vi "Pressure Monitor GUI.vi"(9 "Standalone":bool=TRUE, 10 "Init Data":variant, 11 "My Name":string) -> ()   [LabVIEW 2021]
uses:
  typedefs/CC enum Operation Mode.ctl
  Subsystems/SS typedef cluster Instrument Command Queue Data.ctl
  Subsystems/SS cluster Data Queue type.ctl
  hk-channel-class/HK Item/HK Item.lvclass
  CryoCooler/Cryo Cooler/CryoCoolerAVC/CryoCoolerAVC Command cluster.ctl
  CryoCooler/Cryo Cooler/CryoCoolerAVC/CryoCoolerAVC Command enum.ctl
  Pressure Monitor/Pressure Monitor.lvclass
  typedefs/CC cluster Alarm Data.ctl
  Pressure Monitor/CC cluster Pressure Monitor Settings.ctl
  Pressure Monitor/Lesker Pressure/Lesker Pressure.lvclass
  C:/Development/prime/Prime-RIMAS/Pressure Monitor/Pressure Monitor/Pressure Monitor.lvclass
  Pressure Monitor/Pressure Monitor.lvclass/Pressure Monitor.ctl
  hk-channel-class/HK Item/HK Item.lvclass/HK Item.ctl
  hk-channel-class/HK Item/HK Channel cluster Telemetry Data.ctl
  hk-channel-class/HK Item/HK Channel enum Data Type.ctl
  <vilib>/Utility/error.llb/DialogType.ctl
  Pressure Monitor/Lesker Pressure/Lesker Pressure.lvclass/Lesker Pressure.ctl
  hk-channel-class/HK Item/Write Source.vi
panel:
  in  "Mode":T1
  in  "Tab Control":enum32{"Pressure Monitor", "Engineering", "Log"}(tab)
  in  "Reconnect":bool
  in  "Clear History":bool
  in  "Log Scale":bool=TRUE
  out "Alarm Message":string
  out "Pressure Connected":bool
  out "Alarm":bool
  in  "Status":i32[](listbox) caption="Pressure Monitor"
  out "XY Graph":T2(graph)
  in  "Inst Filament":bool caption="Filament"
  in  "Pump Filament":bool
  in  "Pressure Alarm Level":dbl format="%^_3g"
  in  "Enable Pump Reading?":bool
  in  "Pump Lesker Addr":refnum<visa-resource-name>
  in  "Instrument Lesker Addr":refnum<visa-resource-name>
  in  "CryoCooler Type":u16(ring) items=["Simulation", "PRIME"]
  in  "Close":bool
  out "Log":string
  # "Guage type is 392\nIf the Ion Gauge commands to turn the filament ON and OFF returns a SYNTAX Error, then you\nneed to go to the gauge front panel menu and select:\nFirst TURN IG OFF, then\nSETUP UNIT > IG CNTL > Set to RS485\n\nSee page 30 of the manual"
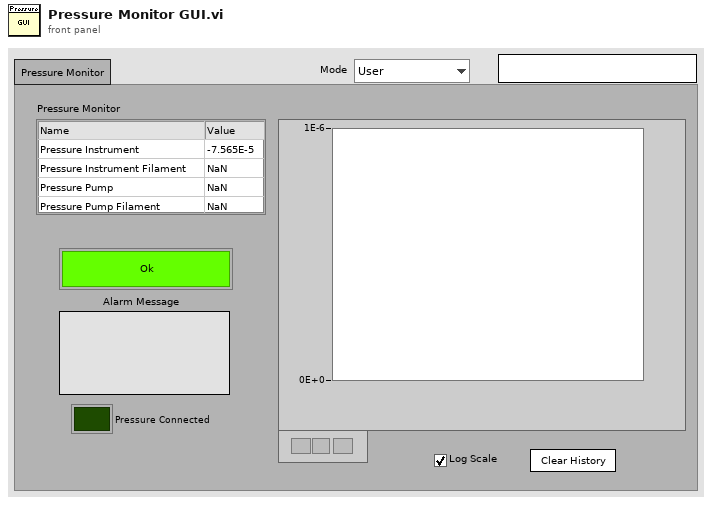
[diagram p1: front panel]
types:
  T1 = typedef "CC enum Operation Mode.ctl" = enum16{"User", "Engineering"}
  T2 = cluster{cluster{"Time Stamp":timestamp, "Numeric":dbl}[]}[]
  T3 = typedef "SS typedef cluster Instrument Command Queue Data.ctl" = cluster{"Cmd":string, "Parameters":variant}
  T4 = typedef "CryoCoolerAVC Command cluster.ctl" = cluster{"Command":T5, "Options":string, "Cryo Idx":i32}
  T5 = typedef "CryoCoolerAVC Command enum.ctl" = u16
  T6 = typedef "CC cluster Alarm Data.ctl" = cluster{"Measured Value":dbl, "Alarm Low":dbl, "Alarm High":dbl, "Message":string, "Source":string}
  T7 = typedef "CC cluster Pressure Monitor Settings.ctl" = cluster{"Lesker Addrs":refnum<visa-resource-name>[], "Enabled?":bool[], "Pressure Alarm Level":dbl, "Filaments":bool[]}
  T8 = cluster{"state":refnum<user-event>, "cmd q":refnum<queue>, "Cmd":T3, "Data Q":refnum<queue>, "error":errorcluster, "next poll":timestamp, "My Name":string, "poll":bool, "Channel List":refnum<class "HK Item.lvclass">[], "Focus Pos":dbl, "Data":dbl[], "Cryo Cmd":T4, "Alarm":bool, "PM Ref":refnum<class "Pressure Monitor.lvclass">, "Alarms":T6[], "Source":string, "Settings":T7}
  T9 = typedef "SS cluster Data Queue type.ctl" = cluster{"Source":string, "Type":string, "Data":variant}
  T10 = typedef "HK Item.lvclass/HK Channel enum Data Type.ctl" = enum16{"Floating Point", "Integer", "Enum", "String", "Waveform", "File"}
  T11 = typedef "HK Item.lvclass/HK Channel cluster Telemetry Data.ctl" = cluster{"Ch Names":string[], "Ch Values":dbl[], "Timestamp":timestamp, "Data Type":T10}
  T12 = typedef "CC cluster Device Index.ctl" = cluster{"Device Type Name":string, "Curr Device Name":string, "All Instances":string[]}
  T13 = cluster{"Select Ch":i32[], "Default Device":string}
  T14 = typedef "HK Item.lvclass/HK Channel Units and Setup.ctl" = cluster{"Unit Type":string, "Units":string, "Configuration":string, "Digits":i32, "Data Type":T10, "Exponential?":bool, "Source":string}
  T15 = cluster{cluster{"Time Stamp":timestamp, "Numeric":dbl}[]}
  T16 = typedef "DialogType.ctl" = u16
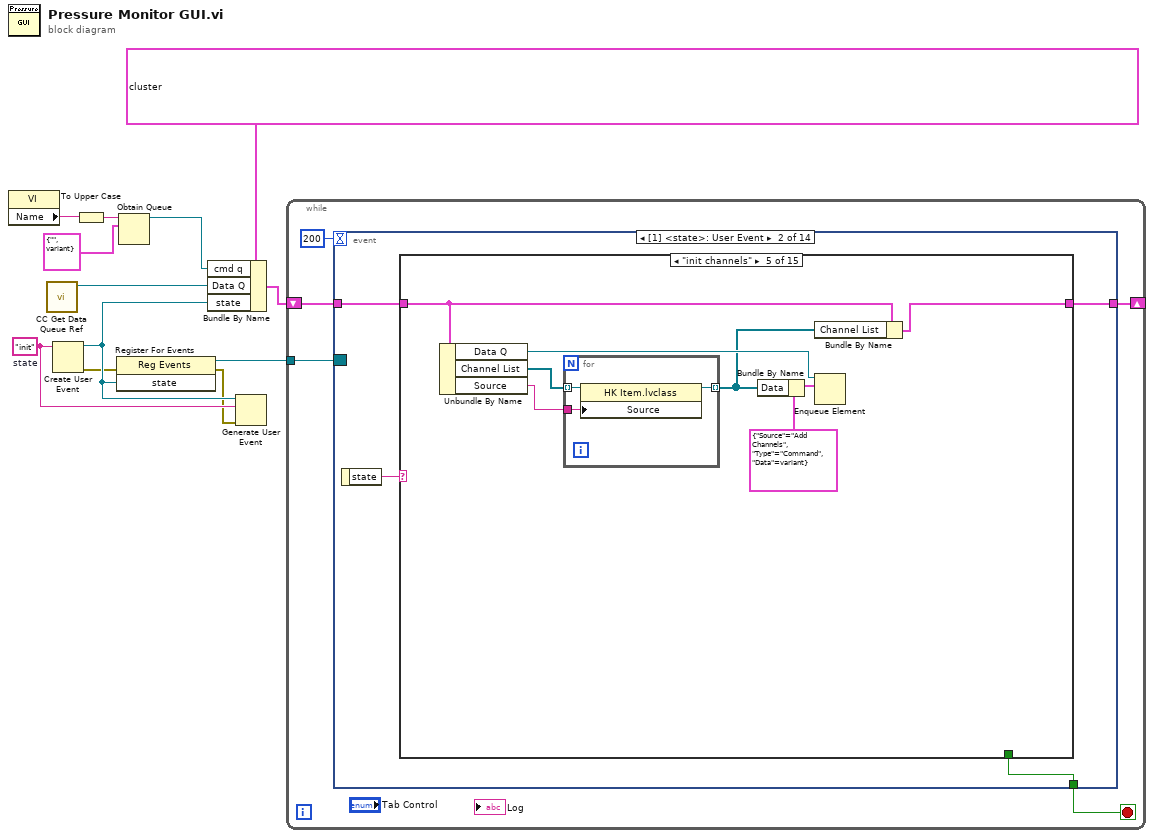
[diagram p0: block diagram]
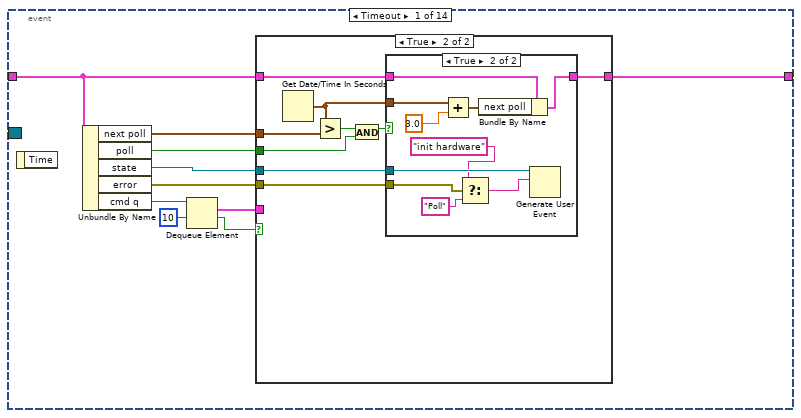
[diagram p2: hidden frame]
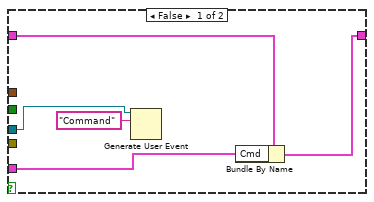
[diagram p3: hidden frame]
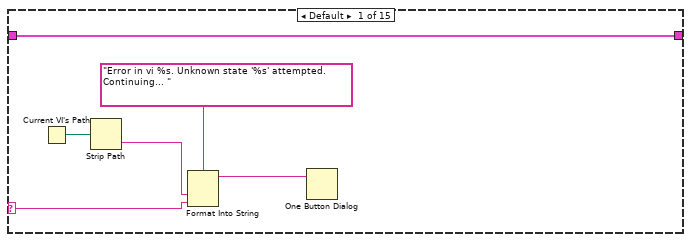
[diagram p5: hidden frame]
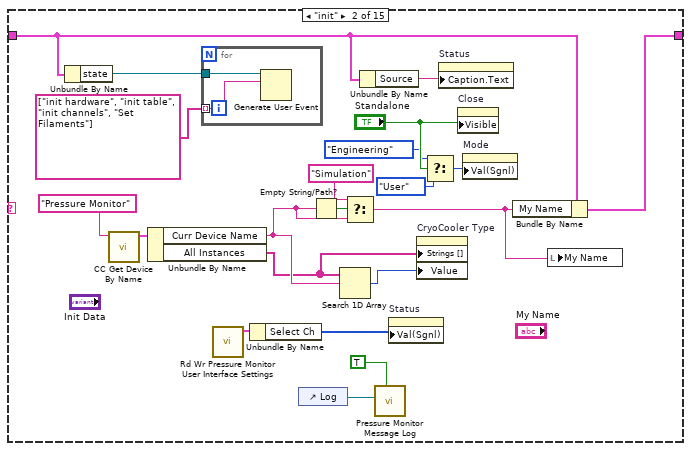
[diagram p6: hidden frame]
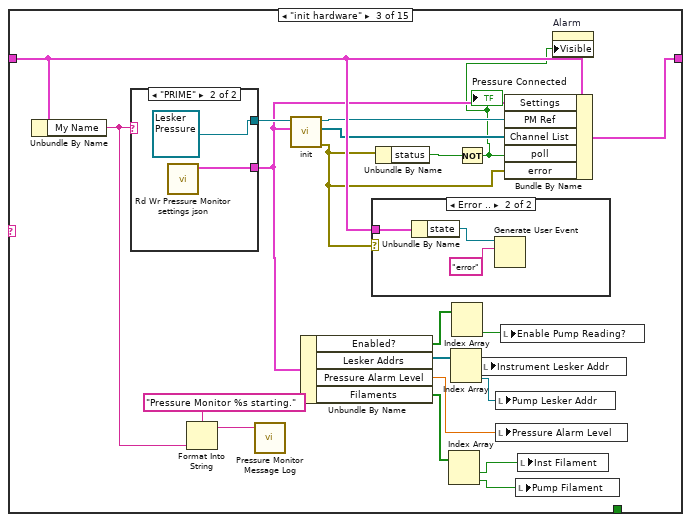
[diagram p7: hidden frame]
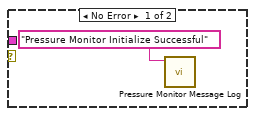
[diagram p8: hidden frame]
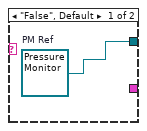
[diagram p9: hidden frame]
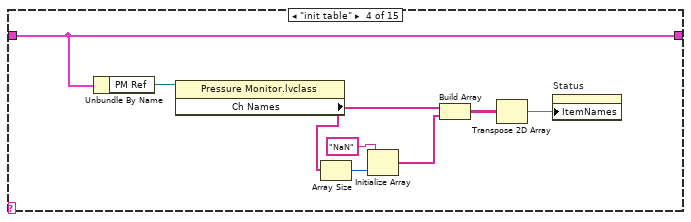
[diagram p10: hidden frame]
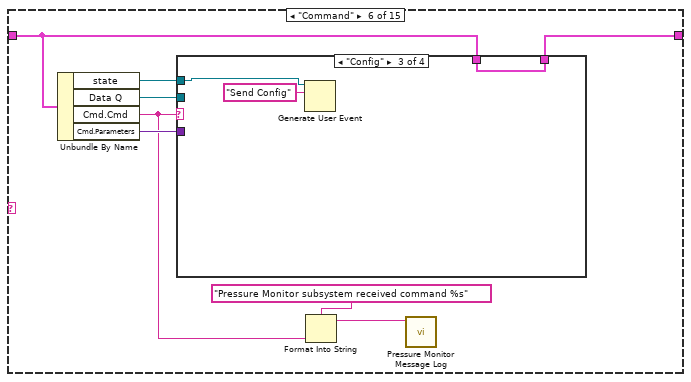
[diagram p11: hidden frame]
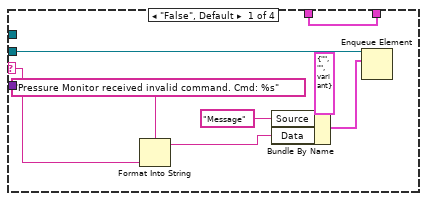
[diagram p12: hidden frame]
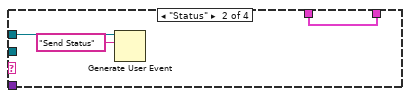
[diagram p13: hidden frame]
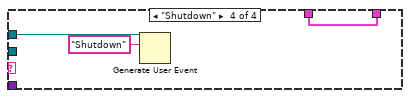
[diagram p14: hidden frame]
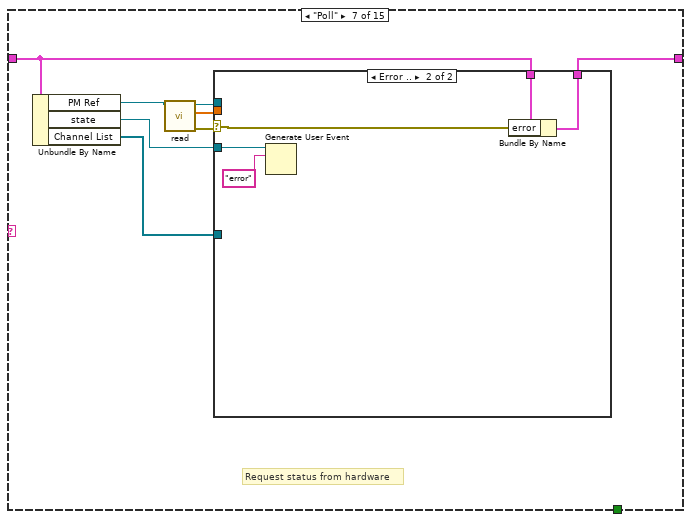
[diagram p15: hidden frame]
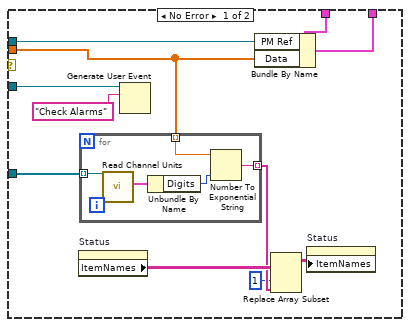
[diagram p16: hidden frame]
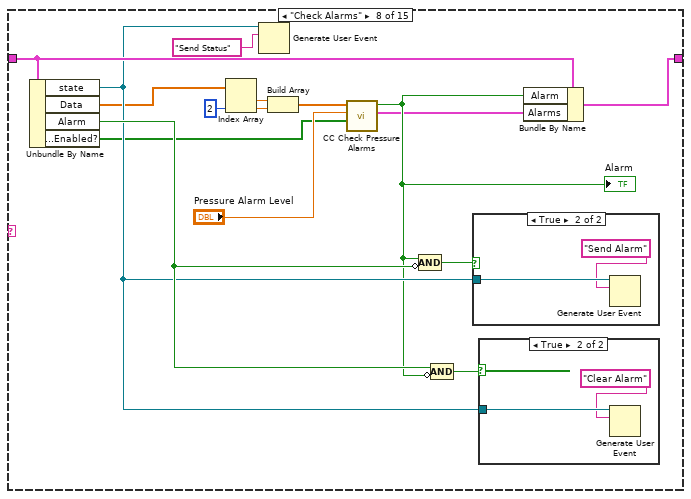
[diagram p17: hidden frame]
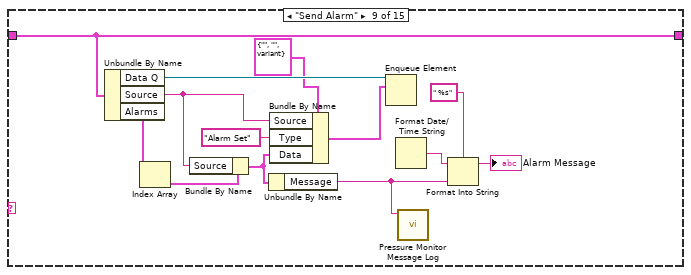
[diagram p20: hidden frame]
diagram:
  w8 = "init"  # state
  n1 = property class="VI"() -> ("Name"=w4:string)  [unwired: 2 in, 2 out]
  n2 = call "CC Get Data Queue Ref.vi"() -> ("Data Q"=w5:refnum<queue>)  [unwired: 10 in, 1 out]
  n3 = Create User Event(user event datatype=w8) -> (user event=w10:refnum<user-event>, error out=w6:errorcluster)  [unwired: 1 in]
  n4 = To Upper Case(1:w4) -> (0:w3:string)
  n5 = register-events(error in=w6, w10) -> (reference out=w9:refnum<event-registration>, error out=w7:errorcluster)  [unwired: 1 in]
  n6 = Obtain Queue(name (unnamed)=w3, element data type=T3 {"Cmd"="", "Parameters"=variant}) -> (queue out=w1:refnum<queue>)  [unwired: 3 in, 2 out]
  n7 = Bundle By Name(cluster=T8 {"state"=refnum, "cmd q"=refnum, "Cmd"={"Cmd"="", "Parameters"=variant}, "Data Q"=refnum, "error"={"status"=FALSE, "code"=0, "source"=""}, "next poll"=timestamp(0 s since 1904-01-01), "My Name"="", "poll"=FALSE, "Channel List"=[], "Focus Pos"=0.0, "Data"=[], "Cryo Cmd"={"Command"=0, "Options"="", "Cryo Idx"=0}, "Alarm"=FALSE, "PM Ref"=refnum, "Alarms"=[], "Source"="Pressure Monitor", "Settings"={"Lesker Addrs"=[], "Enabled?"=[], "Pressure Alarm Level"=0.0001, "Filaments"=[]}}, "cmd q"=w1, "Data Q"=w5, "state"=w10) -> (w11:T8)
  n8 = Generate User Event(user event=w10, event data cluster=w8, error in=w7) -> ()  [unwired: 1 in, 2 out]
  n9 = while {
    tunnel: w9 -> [w17]
    shift-right: [w15] -> _
    shift-left: w11 -> [w16]
    stop <- w14 stop-if-true
    n10 = event shown="[1] <state>: User Event" {
      selector: w17 -> [_ _ _ _ _ _ _ _ _ _ _ _ _ _]
      dyn-events: _ -> [_ _ _ _ _ _ _ _ _ _ _ _ _ _]
      timeout: 200 -> [_ _ _ _ _ _ _ _ _ _ _ _ _ _]
      tunnel: w16 -> [w22 w55 w293 w296 w303 w306 w311 w313 w341 w353 w367 w372 w378 w381]
      tunnel: [w21 w54 w293 w297 w303 w306 w311 w314 w341 w354 w367 w372 w378 w381] -> w15
      tunnel: [_ w53 _ _ _ _ _ _ _ _ _ _ _ _] -> w14
      event Timeout {
        n11 = event-data() -> ()  [unwired: 1 in, 1 out]
        n12 = Unbundle By Name(w22) -> ("next poll"=w20:timestamp, "poll"=w19:bool, "state"=w23:refnum<user-event>, "error"=w18:errorcluster, "cmd q"=w27:refnum<queue>)
        n13 = Dequeue Element(queue=w27, timeout in ms (-1)=10) -> (element=w24:T3, timed out?=w25:bool)  [unwired: 1 in, 2 out]
        n14 = case shown="True" w25 {
          tunnel: w24 -> [w29 _]
          tunnel: w23 -> [w32 w38]
          tunnel: w22 -> [w30 w39]
          tunnel: [w28 w36] -> w21
          tunnel: w20 -> [_ w41]
          tunnel: w19 -> [_ w34]
          tunnel: w18 -> [_ w33]
          frame False {
            n15 = Generate User Event(user event=w32, event data cluster="Command" ("event data")) -> ()  [unwired: 2 in, 2 out]
            n16 = Bundle By Name(cluster=w30, "Cmd"=w29) -> (w28:T8)
          }
          frame True {
            n17 = Get Date/Time In Seconds() -> (seconds since 1Jan1904=w37:timestamp)
            n18 = Greater?(x=w37, y=w41) -> (0:w40:bool)
            n19 = And(x=w40, y=w34) -> (x .and. y?=w35:bool)
            n20 = case shown="True" w35 {
              tunnel: w39 -> [w42 w52]
              tunnel: w38 -> [_ w51]
              tunnel: w37 -> [_ w50]
              tunnel: [w42 w47] -> w36
              tunnel: w33 -> [_ w45]
              frame False {
              }
              frame True {
                n21 = Add(x=w50, y=3.0) -> (x+y=w48:timestamp)
                n22 = Select(t="init hardware" ("event data"), s=w45, f="Poll" ("event data")) -> (s? t:f=w43:string)
                n23 = Bundle By Name(cluster=w52, "next poll"=w48) -> (w47:T8)
                n24 = Generate User Event(user event=w51, event data cluster=w43) -> ()  [unwired: 2 in, 2 out]
              }
            }
          }
        }
      }
      event User Event {
        n25 = event-data() -> ("state"=w56:string)  [unwired: 1 in]
        n26 = case shown="\"init channels\"" w56 {
          selector: w56 -> [w61 _ _ _ _ _ _ _ _ _ _ _ _ _ _]
          tunnel: w55 -> [w57 w64 w103 w121 w122 w136 w164 w200 w219 w226 w243 w248 w259 w265 w289]
          tunnel: [w57 w82 w106 w121 w123 w137 w165 w201 w219 w226 w243 w249 w260 w266 w289] -> w54
          tunnel: [_ _ _ _ _ _ _ _ _ _ _ _ _ _ TRUE] -> w53
          frame Default {
            n27 = Current VI's Path() -> (path=w60:path)
            n28 = Strip Path(path=w60) -> (name=w59:string)  [unwired: 1 out]
            n29 = Format Into String(format string="Error in vi %s. Unknown state '%s' attempted. Continuing... ", w59, w61) -> (resulting string=w58:string)  [unwired: 2 in, 1 out]
            n30 = One Button Dialog(message=w58) -> ()  [unwired: 1 in, 1 out]
          }
          frame "init" {
            n31 = Unbundle By Name(w64) -> ("state"=w81:refnum<user-event>)
            n32 = call "CC Get Device By Name.vi"("Device Type"="Pressure Monitor") -> ("Device"=w76:T12)  [unwired: 8 in, 2 out]
            n33 = Unbundle By Name(w76) -> ("Curr Device Name"=w75:string, "All Instances"=w74:string[])
            n34 = for {
              tunnel: w81 -> [w85]
              tunnel: string[] ["init hardware", "init table", "init channels", "Set Filaments"] -> [w84] mode=indexing
              n35 = Generate User Event(user event=w85, event data cluster=w84) -> ()  [unwired: 2 in, 2 out]
            }
            n36 = call "Rd Wr Pressure Monitor User Interface Settings.vi"() -> ("Settings"=w66:T13)  [unwired: 10 in, 1 out]
            n37 = Unbundle By Name(w66) -> ("Select Ch"=w65:i32[])
            n38 = control-ref of="Log"() -> (w69:refnum<vi>)
            n39 = Empty String/Path?(string/path=w75) -> (empty?=w83:bool)
            n40 = Search 1D Array(1D array=w74, element=w75) -> (index of element=w79:i32)  [unwired: 1 in]
            n41 = Select(t="Simulation", s=w83, f=w75) -> (s? t:f=w67:string)
            n42 = Unbundle By Name(w64) -> ("Source"=w63:string)
            n43 = call "Pressure Monitor Message Log.vi"("init?"=TRUE, "Log Ref"=w69) -> ()  [unwired: 8 in, 2 out]
            n44 = property on="Status" class="MCListbox (strict)"("Val(Sgnl)"=w65) -> ()  [unwired: 2 in, 2 out]
            n45 = property on="CryoCooler Type" class="Ring (strict)"("Strings []"=w74, "Value"=w79) -> ()  [unwired: 2 in, 2 out]
            n46 = Select(t=CC_enum_Operation_Mode."Engineering" ("Mode"), s="Standalone", f=CC_enum_Operation_Mode."User" ("Mode")) -> (s? t:f=w70:T1)
            n47 = property on="Status" class="MCListbox (strict)"("Caption.Text"=w63) -> ()  [unwired: 2 in, 2 out]
            n48 = property on="Close" class="Bool"("Visible"="Standalone") -> ()  [unwired: 2 in, 2 out]
            n49 = property on="Mode" class="Enum (strict)"("Val(Sgnl)"=w70) -> ()  [unwired: 2 in, 2 out]
            n50 = Bundle By Name(cluster=w64, "My Name"=w67) -> (w82:T8)
            n51 = local write "My Name"(w67) -> ()
          }
          frame "init hardware" {
            n52 = Unbundle By Name(w103) -> ("My Name"=w105:string)
            n53 = case shown="\"PRIME\"" w105 {
              tunnel: [w111 refnum<class "Lesker Pressure.lvclass"> refnum ("Lesker Pressure.lvclass")] -> w101
              tunnel: [_ w113] -> w91
              frame "False", Default {
                w111 = refnum<class "Pressure Monitor.lvclass"> refnum  # PM Ref
              }
              frame "PRIME" {
                n54 = call "Rd Wr Pressure Monitor settings json.vi"() -> ("Pressur Monitor Settings"=w113:T7)  [unwired: 10 in, 1 out]
              }
            }
            n55 = Format Into String(format string="Pressure Monitor %s starting.", w105) -> (resulting string=w102:string)  [unwired: 2 in, 1 out]
            n56 = call "Pressure Monitor Message Log.vi"("String in"=w102) -> ()  [unwired: 9 in, 2 out]
            n57 = call-dynamic "init.vi"("Init Data"=w91, "Pressure Monitor in"=w101) -> ("error out"=w98:errorcluster, "Channel List"=w99:refnum<class "HK Item.lvclass">[], "Pressure Monitor out"=w100:refnum<class "Pressure Monitor.lvclass">)  [unwired: 7 in]
            n58 = Unbundle By Name(w91) -> ("Enabled?"=w93:bool[], "Lesker Addrs"=w97:refnum<visa-resource-name>[], "Pressure Alarm Level"=w94:dbl, "Filaments"=w90:bool[])
            n59 = case shown="Error .." w98 {
              tunnel: w103 -> [_ w110]
              frame No Error {
                n60 = call "Pressure Monitor Message Log.vi"("String in"="Pressure Monitor Initialize Successful") -> ()  [unwired: 9 in, 2 out]
              }
              frame Error {
                n61 = Unbundle By Name(w110) -> ("state"=w109:refnum<user-event>)
                n62 = Generate User Event(user event=w109, event data cluster="error" ("event data")) -> ()  [unwired: 2 in, 2 out]
              }
            }
            n63 = Unbundle By Name(w98) -> ("status"=w87:bool)
            n64 = Index Array(array=w90) -> (element #1=w89:bool, element #2=w88:bool)  [unwired: 2 in]
            n65 = Index Array(array=w97) -> (element #1=w96:refnum<visa-resource-name>, element #2=w95:refnum<visa-resource-name>)  [unwired: 2 in]
            n66 = Index Array(array=w93) -> (element #2=w92:bool)  [unwired: 2 in, 1 out]
            n67 = Not(x=w87) -> (.not. x?=w86:bool)
            "Pressure Connected" <- w86
            n68 = local write "Instrument Lesker Addr"(w96) -> ()
            n69 = local write "Pump Lesker Addr"(w95) -> ()
            n70 = local write "Pressure Alarm Level"(w94) -> ()
            n71 = local write "Enable Pump Reading?"(w92) -> ()
            n72 = Bundle By Name(cluster=w103, "Settings"=w91, "PM Ref"=w100, "Channel List"=w99, "poll"=w86, "error"=w98) -> (w106:T8)
            n73 = local write "Pump Filament"(w88) -> ()
            n74 = local write "Inst Filament"(w89) -> ()
            n75 = property on="Alarm" class="Bool (strict)"("Visible"=w86) -> ()  [unwired: 2 in, 2 out]
          }
          frame "init table" {
            n76 = Unbundle By Name(w121) -> ("PM Ref"=w120:refnum<class "Pressure Monitor.lvclass">)
            n77 = property class="Pressure Monitor.lvclass"(reference=w120) -> ("Ch Names"=w117:string[])  [unwired: 1 in, 2 out]
            n78 = Array Size(array=w117) -> (size(s)=w119:i32)
            n79 = Initialize Array("NaN", w119) -> (w118:string[])
            n80 = Build Array(w117, w118) -> (w115:string[][])
            n81 = Transpose 2D Array(2D array=w115) -> (transposed array=w114:string[][])
            n82 = property on="Status" class="MCListbox (strict)"("ItemNames"=w114) -> ()  [unwired: 2 in, 2 out]
          }
          frame "init channels" {
            n83 = Unbundle By Name(w122) -> ("Data Q"=w127:refnum<queue>, "Channel List"=w126:refnum<class "HK Item.lvclass">[], "Source"=w125:string)
            n84 = for {
              tunnel: w126 -> [w132] mode=indexing
              tunnel: [w131] -> w124 mode=indexing
              tunnel: w125 -> [w130]
              n85 = property class="HK Item.lvclass"(reference=w132, "Source"=w130) -> (reference out=w131:refnum<class "HK Item.lvclass">)  [unwired: 1 in, 1 out]
            }
            n86 = Bundle By Name(cluster=T9 {"Source"="Add Channels", "Type"="Command", "Data"=variant} ("element"), "Data"=w124) -> (w129:T9)
            n87 = Bundle By Name(cluster=w122, "Channel List"=w124) -> (w123:T8)
            n88 = Enqueue Element(queue=w127, element=w129) -> ()  [unwired: 2 in, 3 out]
          }
          frame "Command" {
            n89 = Unbundle By Name(w136) -> ("state"=w138:refnum<user-event>, "Data Q"=w140:refnum<queue>, "Cmd.Cmd"=w134:string, "Cmd.Parameters"=w139:variant)
            n90 = case shown="\"Config\"" w134 {
              selector: w134 -> [w142 _ _ _]
              tunnel: w140 -> [w148 _ _ _]
              tunnel: w139 -> [_ _ _ _]
              tunnel: w138 -> [_ w151 w153 w157]
              tunnel: w136 -> [w141 w149 w152 w155]
              tunnel: [w141 w149 w152 w155] -> w137
              frame "False", Default {
                n91 = Format Into String(format string="Pressure Monitor received invalid command. Cmd: %s", w142) -> (resulting string=w144:string)  [unwired: 2 in, 1 out]
                n92 = Bundle By Name(cluster=T9 {"Source"="", "Type"="", "Data"=variant} ("element"), "Source"="Message" ("Data Type"), "Data"=w144) -> (w143:T9)
                n93 = Enqueue Element(queue=w148, element=w143) -> ()  [unwired: 2 in, 3 out]
              }
              frame "Status" {
                n94 = Generate User Event(user event=w151, event data cluster="Send Status" ("event data")) -> ()  [unwired: 2 in, 2 out]
              }
              frame "Config" {
                n95 = Generate User Event(user event=w153, event data cluster="Send Config" ("event data")) -> ()  [unwired: 2 in, 2 out]
              }
              frame "Shutdown" {
                n96 = Generate User Event(user event=w157, event data cluster="Shutdown" ("event data")) -> ()  [unwired: 2 in, 2 out]
              }
            }
            n97 = Format Into String(format string="Pressure Monitor subsystem received command %s", w134) -> (resulting string=w133:string)  [unwired: 2 in, 1 out]
            n98 = call "Pressure Monitor Message Log.vi"("String in"=w133) -> ()  [unwired: 9 in, 2 out]
          }
          frame "Poll" {
            # "Request status from hardware"
            n99 = Unbundle By Name(w164) -> ("PM Ref"=w161:refnum<class "Pressure Monitor.lvclass">, "state"=w163:refnum<user-event>, "Channel List"=w162:refnum<class "HK Item.lvclass">[])
            n100 = call-dynamic "read.vi"("Pressure Monitor in"=w161) -> ("error out"=w158:errorcluster, "Data"=w159:dbl[], "Pressure Monitor out"=w160:refnum<class "Pressure Monitor.lvclass">)  [unwired: 8 in]
            n101 = case shown="Error .." w158 {
              selector: w158 -> [_ w183]
              tunnel: [w176 w182] -> w165
              tunnel: w164 -> [w175 w184]
              tunnel: w163 -> [w174 w186]
              tunnel: w160 -> [w172 _]
              tunnel: w162 -> [w171 _]
              tunnel: w159 -> [w170 _]
              frame No Error {
                n102 = property on="Status" class="MCListbox (strict)"() -> ("ItemNames"=w169:string[][])  [unwired: 2 in, 2 out]
                n103 = for {
                  tunnel: w171 -> [w181] mode=indexing
                  tunnel: w170 -> [w178] mode=indexing
                  tunnel: [w177] -> w168 mode=indexing
                  n104 = call "Read Channel Units.vi"("HK Item in"=w181) -> ("Channel Setup"=w180:T14)  [unwired: 8 in, 2 out]
                  n105 = Unbundle By Name(w180) -> ("Digits"=w179:i32)
                  n106 = Number To Exponential String(number=w178, precision (6)=w179) -> (E-format string=w177:string)  [unwired: 2 in]
                }
                n107 = Generate User Event(user event=w174, event data cluster="Check Alarms" ("event data")) -> ()  [unwired: 2 in, 2 out]
                n108 = Bundle By Name(cluster=w175, "PM Ref"=w172, "Data"=w170) -> (w176:T8)
                n109 = Replace Array Subset(array=w169, new element=w168, index (col)=1 ("disabled index (col)")) -> (w166:string[][])  [unwired: 1 in]
                n110 = property on="Status" class="MCListbox (strict)"("ItemNames"=w166) -> ()  [unwired: 2 in, 2 out]
              }
              frame Error {
                n111 = Generate User Event(user event=w186, event data cluster="error" ("event data")) -> ()  [unwired: 2 in, 2 out]
                n112 = Bundle By Name(cluster=w184, "error"=w183) -> (w182:T8)
              }
            }
          }
          frame "Check Alarms" {
            n113 = Unbundle By Name(w200) -> ("state"=w196:refnum<user-event>, "Data"=w191:dbl[], "Alarm"=w198:bool, "Settings.Enabled?"=w192:bool[])
            n114 = Index Array(array=w191, index #2=2 ("index")) -> (element #1=w188:dbl, element #2=w189:dbl)  [unwired: 1 in]
            n115 = Generate User Event(user event=w196, event data cluster="Send Status" ("event data")) -> ()  [unwired: 2 in, 2 out]
            n116 = Build Array(w188, w189) -> (w187:dbl[])
            n117 = call "CC Check Pressure Alarms.vi"("Enabled?"=w192, "Pressure Alarm Level"="Pressure Alarm Level", "Presssure Data"=w187) -> ("Alarms"=w193:T6[], "Alarm"=w194:bool)  [unwired: 6 in, 1 out]
            "Alarm" <- w194
            n118 = Compound Arithmetic op=AND(w194, invert w198) -> (w199:bool)
            n119 = Compound Arithmetic op=AND(w198, invert w194) -> (w197:bool)
            n120 = case shown="True" w199 {
              tunnel: w196 -> [_ w206]
              frame False {
              }
              frame True {
                n121 = Generate User Event(user event=w206, event data cluster="Send Alarm" ("event data")) -> ()  [unwired: 2 in, 2 out]
              }
            }
            n122 = case shown="True" w197 {
              tunnel: w196 -> [_ w204]
              frame False {
              }
              frame True {
                n123 = Generate User Event(user event=w204, event data cluster="Clear Alarm" ("event data")) -> ()  [unwired: 2 in, 2 out]
              }
            }
            n124 = Bundle By Name(cluster=w200, "Alarm"=w194, "Alarms"=w193) -> (w201:T8)
          }
          frame "Send Alarm" {
            n125 = Unbundle By Name(w219) -> ("Data Q"=w218:refnum<queue>, "Source"=w207:string, "Alarms"=w215:T6[])
            n126 = Index Array(array=w215) -> (element=w209:T6)  [unwired: 1 in]
            n127 = Bundle By Name(cluster=w209, "Source"=w207) -> (w208:T6)
            n128 = Unbundle By Name(w208) -> ("Message"=w212:string)
            n129 = Bundle By Name(cluster=T9 {"Source"="", "Type"="", "Data"=variant} ("element"), "Source"=w207, "Type"="Alarm Set", "Data"=w208) -> (w214:T9)
            n130 = Enqueue Element(queue=w218, element=w214) -> ()  [unwired: 2 in, 3 out]
            n131 = Format Date/Time String() -> (date/time string=w210:string)  [unwired: 3 in]
            n132 = call "Pressure Monitor Message Log.vi"("String in"=w212) -> ()  [unwired: 9 in, 2 out]
            n133 = Format Into String(format string=" %s", initial string=w210, w212) -> (resulting string=→"Alarm Message":string)  [unwired: 1 in, 1 out]
          }
          frame "Clear Alarm" {
            w221 = "Alarm condition cleared." ("String in")
            n134 = Unbundle By Name(w226) -> ("Data Q"=w225:refnum<queue>, "Source"=w222:string)
            n135 = Bundle By Name(cluster=T9 {"Source"="", "Type"="", "Data"=variant} ("element"), "Source"=w222, "Type"="Alarm Clear") -> (w220:T9)
            n136 = Enqueue Element(queue=w225, element=w220) -> ()  [unwired: 2 in, 3 out]
            n137 = call "Pressure Monitor Message Log.vi"("String in"=w221) -> ()  [unwired: 9 in, 2 out]
            n138 = local write "Alarm Message"(w221) -> ()
          }
          frame "Send Status" {
            n139 = Unbundle By Name(w243) -> ("Data Q"=w242:refnum<queue>, "Source"=w227:string, "PM Ref"=w229:refnum<class "Pressure Monitor.lvclass">, "Data"=w234:dbl[])
            n140 = Get Date/Time In Seconds() -> (seconds since 1Jan1904=w235:timestamp)
            n141 = call "Read Ch Names.vi"("Pressure Monitor in"=w229) -> ("Ch Names"=w228:string[])  [unwired: 8 in, 2 out]
            n142 = Bundle(cluster=T11 {"Ch Names"=[], "Ch Values"=[], "Timestamp"=timestamp(0 s since 1904-01-01), "Data Type"=enum."Floating Point"}, "Ch Names"=w228, "Ch Values"=w234, "Timestamp"=w235, "Data Type"=HK_Channel_enum_Data_Type."Floating Point") -> (w237:T11)
            n143 = call "CC Pressure Monitor Data buffer.vi"("Write?"=TRUE, "Data"=w234, "Time Stamp"=w235) -> ("XY Graph"=w231:T2)  [unwired: 7 in, 1 out]
            n144 = for {
              tunnel: "Status" -> [w245] mode=indexing
              tunnel: w231 -> [w246]
              tunnel: [w244] -> w230 mode=indexing
              n145 = Index Array(array=w246, index=w245) -> (element=w244:T15)
            }
            "XY Graph" <- w230
            n146 = Bundle By Name(cluster=T9 {"Source"="", "Type"="", "Data"=variant} ("element"), "Source"=w227, "Type"="Floating Point" ("Data Type"), "Data"=w237) -> (w239:T9)
            n147 = Enqueue Element(queue=w242, element=w239) -> ()  [unwired: 2 in, 3 out]
          }
          frame "Set Filaments" {
            n148 = Unbundle By Name(w248) -> ("PM Ref"=w251:refnum<class "Pressure Monitor.lvclass">, "Settings.Filaments"=w247:bool[])
            n149 = for {
              shift-right: [w254] -> w250
              shift-left: w251 -> [w255]
              tunnel: w247 -> [w253] mode=indexing
              i -> [w252]
              n150 = call-dynamic "Filament Control.vi"("Filament"=w253, "Filament ID"=w252, "Pressure Monitor in"=w255) -> ("Pressure Monitor out"=w254:refnum<class "Pressure Monitor.lvclass">)  [unwired: 7 in, 1 out]
            }
            n151 = Bundle By Name(cluster=w248, "PM Ref"=w250) -> (w249:T8)
          }
          frame "Reinit" {
            n152 = Unbundle By Name(w259) -> ("PM Ref"=w258:refnum<class "Pressure Monitor.lvclass">, "state"=w262:refnum<user-event>)
            n153 = call-dynamic "close.vi"("Pressure Monitor in"=w258) -> ("error out"=w256:errorcluster, "Pressure Monitor out"=w257:refnum<class "Pressure Monitor.lvclass">)  [unwired: 9 in]
            n154 = Generate User Event(user event=w262, event data cluster="init hardware" ("event data")) -> ()  [unwired: 2 in, 2 out]
            n155 = call <vilib>:"Clear Errors.vi"("error in (no error)"=w256) -> ()  [unwired: 5 in, 2 out]
            n156 = Bundle By Name(cluster=w259, "PM Ref"=w257) -> (w260:T8)
          }
          frame "error" {
            w263 = FALSE ("Pressure Connected")
            w270 = T16 0 items=["no dialog", "OK message", "continue or stop message", "OK message + warnings", "continue/stop + warnings"] ("type of dialog (OK msg:1)")
            # "Wait 3 minutes before trying again"
            n157 = Unbundle By Name(w265) -> ("My Name"=w274:string, "error"=w281:errorcluster, "error.code"=w284:i32, "error.source"=w282:string, "Data Q"=w272:refnum<queue>)
            n158 = local write "Pressure Connected"(w263) -> ()
            n159 = property on="Alarm" class="Bool (strict)"("Visible"=w263) -> ()  [unwired: 2 in, 2 out]
            n160 = property on="Reconnect" class="Bool"("Visible"=TRUE) -> ()  [unwired: 2 in, 2 out]
            n161 = call <vilib>:"Simple Error Handler.vi"("type of dialog (OK msg:1)"=w270, "error in (no error)"=w281) -> ("message"=w280:string)  [unwired: 3 in, 4 out]
            n162 = Bundle By Name(cluster=T6 {"Measured Value"=0.0, "Alarm Low"=0.0, "Alarm High"=0.0, "Message"="", "Source"=""} ("element"), "Source"=w274, "Message"="Pressure Monitor Initialization Error. Check Communications port.") -> (w275:T6)
            n163 = Format Into String(format string="Error from Pressure Monitors \"%s\". Error # %d, Error Source: %s, Error message \"%s\"", w274, w284, w282, w280) -> (resulting string=w279:string)  [unwired: 2 in, 1 out]
            n164 = Bundle By Name(cluster=T9 {"Source"="", "Type"="", "Data"=variant} ("element"), "Source"=w274, "Type"="Alarm Set", "Data"=w275) -> (w271:T9)
            n165 = call "Pressure Monitor Message Log.vi"("String in"=w279) -> ()  [unwired: 9 in, 2 out]
            n166 = Get Date/Time In Seconds() -> (seconds since 1Jan1904=w269:timestamp)
            n167 = Add(x=w269, y=180.0) -> (x+y=w267:timestamp)
            n168 = Enqueue Element(queue=w272, element=w271) -> ()  [unwired: 2 in, 3 out]
            n169 = Bundle By Name(cluster=w265, "next poll"=w267) -> (w266:T8)
          }
          frame "Shutdown" {
            n170 = Unbundle By Name(w289) -> ("Data Q"=w288:refnum<queue>, "PM Ref"=w286:refnum<class "Pressure Monitor.lvclass">)
            n171 = Release Queue(queue=w288) -> ()  [unwired: 2 in, 3 out]
            n172 = call-dynamic "close.vi"("Pressure Monitor in"=w286) -> ("error out"=w285:errorcluster)  [unwired: 9 in, 1 out]
            n173 = call "Pressure Monitor Message Log.vi"("String in"="Pressure Monitor shutting down.") -> ()  [unwired: 9 in, 2 out]
            n174 = call <vilib>:"Clear Errors.vi"("error in (no error)"=w285) -> ()  [unwired: 5 in, 2 out]
          }
        }
      }
      event "Reconnect": Value Change {
        n175 = event-data() -> ()  [unwired: 1 in, 6 out]
        n176 = Unbundle By Name(w293) -> ("state"=w292:refnum<user-event>)
        n177 = Generate User Event(user event=w292, event data cluster="init hardware" ("event data")) -> ()  [unwired: 2 in, 2 out]
      }
      event "Pump Filament", "Inst Filament": Value Change {
        n178 = event-data() -> ()  [unwired: 1 in, 6 out]
        n179 = Unbundle By Name(w296) -> ("state"=w295:refnum<user-event>)
        n180 = Generate User Event(user event=w295, event data cluster="Set Filaments" ("event data")) -> ()  [unwired: 2 in, 2 out]
        n181 = Build Array("Inst Filament", "Pump Filament") -> (w298:bool[])
        n182 = Bundle By Name(cluster=w296, "Settings.Filaments"=w298) -> (w297:T8)
      }
      event "Log Scale": Value Change {
        n183 = event-data() -> ()  [unwired: 1 in, 6 out]
        n184 = Boolean To (0,1)(Boolean="Log Scale") -> (0, 1=w301:i16)
        n185 = property on="XY Graph" class="XYGraph (strict)"("YScale.Mapping Mode"=w301) -> ()  [unwired: 2 in, 2 out]
      }
      event "Clear History": Value Change {
        n186 = event-data() -> ()  [unwired: 1 in, 6 out]
        n187 = call "CC Pressure Monitor Data buffer.vi"("Clear"=TRUE, "Write?"=FALSE) -> ()  [unwired: 8 in, 2 out]
      }
      event "Pressure Alarm Level": Value Change {
        n188 = event-data() -> ("NewVal"=w309:dbl)  [unwired: 1 in]
        n189 = call "Rd Wr Pressure Monitor settings json.vi"() -> ("Pressur Monitor Settings"=w310:T7)  [unwired: 10 in, 1 out]
        n190 = Bundle By Name(cluster=w310, "Pressure Alarm Level"=w309) -> (w308:T7)
        n191 = call "Rd Wr Pressure Monitor settings json.vi"("Write? (F:Read)"=TRUE, "Pressur Monitor Settings"=w308) -> ()  [unwired: 8 in, 2 out]
      }
      event "Enable Pump Reading?": Value Change {
        n192 = event-data() -> ()  [unwired: 1 in, 6 out]
        n193 = Unbundle By Name(w313) -> ("My Name"=w312:string, "PM Ref"=w316:refnum<class "Pressure Monitor.lvclass">)
        n194 = case shown="\"PRIME\"" w312 {
          tunnel: w316 -> [_ w331]
          tunnel: "Enable Pump Reading?" -> [_ w326]
          tunnel: [w317 w323] -> w314
          tunnel: w313 -> [w317 w322]
          frame "False", Default {
          }
          frame "PRIME" {
            n195 = To More Specific Class(target class=refnum<class "Lesker Pressure.lvclass"> refnum ("Lesker Pressure.lvclass"), reference=w331) -> (specific class reference=w330:refnum<class "Lesker Pressure.lvclass">)  [unwired: 1 in, 1 out]
            n196 = call "Rd Wr Pressure Monitor settings json.vi"() -> ("Pressur Monitor Settings"=w321:T7)  [unwired: 10 in, 1 out]
            n197 = call "Read Enabled_.vi"("Lesker Pressure in"=w330) -> ("Enabled?"=w328:bool[], "Lesker Pressure out"=w325:refnum<class "Lesker Pressure.lvclass">)  [unwired: 8 in, 1 out]
            n198 = Replace Array Subset(array=w328, new element=w326, index=1) -> (w319:bool[])
            n199 = Bundle By Name(cluster=w321, "Enabled?"=w319) -> (w318:T7)
            n200 = call "Write Enabled_.vi"("Enabled?"=w319, "Lesker Pressure in"=w325) -> ("Lesker Pressure out"=w324:refnum<class "Lesker Pressure.lvclass">)  [unwired: 8 in, 1 out]
            n201 = Bundle By Name(cluster=w322, "PM Ref"=w324, "Settings"=w318) -> (w323:T8)
            n202 = call "Rd Wr Pressure Monitor settings json.vi"("Write? (F:Read)"=TRUE, "Pressur Monitor Settings"=w318) -> ()  [unwired: 8 in, 2 out]
          }
        }
      }
      event "Status": Value Change {
        n203 = event-data() -> ("NewVal"=w336:i32[])  [unwired: 1 in]
        n204 = call "CC Pressure Monitor Data buffer.vi"() -> ("XY Graph"=w340:T2)  [unwired: 10 in, 1 out]
        n205 = call "Rd Wr Pressure Monitor User Interface Settings.vi"() -> ("Settings"=w337:T13)  [unwired: 10 in, 1 out]
        n206 = for {
          tunnel: w336 -> [w343] mode=indexing
          tunnel: w340 -> [w344]
          tunnel: [w342] -> w339 mode=indexing
          n207 = Index Array(array=w344, index=w343) -> (element=w342:T15)
        }
        n208 = Bundle By Name(cluster=w337, "Select Ch"=w336) -> (w335:T13)
        n209 = Unbundle By Name(w341) -> ("PM Ref"=w333:refnum<class "Pressure Monitor.lvclass">)
        n210 = call "Read Ch Names.vi"("Pressure Monitor in"=w333) -> ("Ch Names"=w332:string[])  [unwired: 8 in, 2 out]
        n211 = call "Rd Wr Pressure Monitor User Interface Settings.vi"("Write? (F:Read)"=TRUE, "Settings"=w335) -> ()  [unwired: 8 in, 2 out]
        n212 = property on="XY Graph" class="XYGraph (strict)"("Value"=w339) -> (error out=w338:errorcluster)  [unwired: 2 in, 1 out]
        n213 = for {
          N -> [w346]
          tunnel: w336 -> [w349] mode=indexing
          tunnel: w332 -> [w350]
          tunnel: w338 -> [w345]
          i -> [w348]
          n214 = Index Array(array=w350, index=w349) -> (element=w347:string)
          n215 = property on="XY Graph" class="XYGraph (strict)"(error in=w345, "Active Plot"=w348, "Plot.Plot Name"=w347, "LegNumRows"=w346) -> ()  [unwired: 1 in, 2 out]
        }
      }
      event "CryoCooler Type": Value Change {
        n216 = event-data() -> ("CtlRef"=w358:refnum<vi>)  [unwired: 1 in, 5 out]
        n217 = property class="Ring (strict)"(reference=w358) -> ("Strings []"=w357:string[])  [unwired: 1 in, 2 out]
        n218 = Unbundle By Name(w353) -> ("state"=w352:refnum<user-event>)
        n219 = Generate User Event(user event=w352, event data cluster="Reinit" ("event data")) -> ()  [unwired: 2 in, 2 out]
        n220 = Index Array(array=w357, index="CryoCooler Type") -> (element=w355:string)
        n221 = Bundle By Name(cluster=w353, "My Name"=w355) -> (w354:T8)
      }
      event "Instrument Lesker Addr", "Pump Lesker Addr": Value Change {
        n222 = event-data() -> ()  [unwired: 1 in, 6 out]
        n223 = call "Rd Wr Pressure Monitor settings json.vi"("Write? (F:Read)"=FALSE) -> ("Pressur Monitor Settings"=w363:T7)  [unwired: 9 in, 1 out]
        n224 = Unbundle By Name(w367) -> ("state"=w366:refnum<user-event>)
        n225 = Build Array("Instrument Lesker Addr", "Pump Lesker Addr") -> (w359:refnum<visa-resource-name>[])
        n226 = Generate User Event(user event=w366, event data cluster="Reinit" ("event data")) -> ()  [unwired: 2 in, 2 out]
        n227 = Bundle By Name(cluster=w363, "Lesker Addrs"=w359) -> (w362:T7)
        n228 = call "Rd Wr Pressure Monitor settings json.vi"("Write? (F:Read)"=TRUE, "Pressur Monitor Settings"=w362) -> ()  [unwired: 8 in, 2 out]
      }
      event Value Change {
        n229 = event-data() -> ()  [unwired: 1 in, 6 out]
        n230 = case shown="\"User\", Default" "Mode" {
          tunnel: [bool[] [TRUE, FALSE, FALSE] bool[] [TRUE, TRUE, TRUE]] -> w369
          frame "User", Default {
          }
          frame "Engineering" {
          }
        }
        n231 = property on="Tab Control" class="TabCtl (strict)"() -> ("Pages"=w370:refnum<vi>[])  [unwired: 2 in, 2 out]
        n232 = for {
          tunnel: w370 -> [w374] mode=indexing
          tunnel: w369 -> [w373] mode=indexing
          n233 = property class="Page"(reference=w374, "PageVis"=w373) -> ()  [unwired: 1 in, 2 out]
        }
      }
      event "Standalone": Value Change {
        n234 = event-data() -> ("NewVal"=w377:bool)  [unwired: 1 in, 5 out]
        n235 = property on="Close" class="Bool"("Visible"=w377) -> ()  [unwired: 2 in, 2 out]
      }
      event "Close": Value Change {
        n236 = event-data() -> ()  [unwired: 1 in, 2 out]
        n237 = Unbundle By Name(w381) -> ("state"=w380:refnum<user-event>)
        n238 = Generate User Event(user event=w380, event data cluster="Shutdown" ("event data")) -> ()  [unwired: 2 in, 2 out]
      }
    }
  }
